vi "XML_AppendSubContent.vi"(10 "string":string, 11 "XML String":string) -> (3 "delimited string":string)   [LabVIEW 2014]
uses:
  <userlib>/_OpenG.lib/string/string.llb/Trim Whitespace (String Array)__ogtk.vi
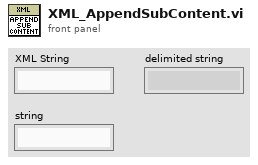
[diagram p1: front panel]
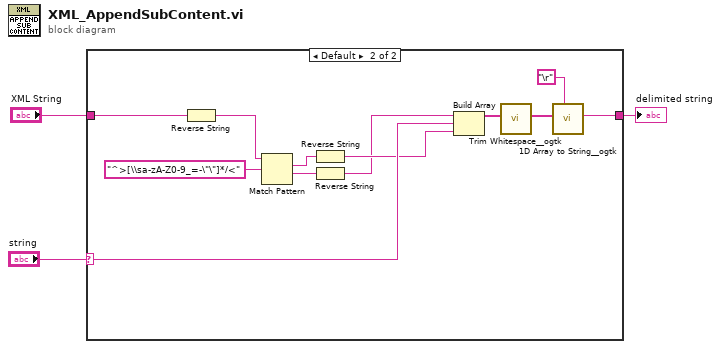
[diagram p0: block diagram]
diagram:
  n1 = case shown="Default" "string" {
    selector: "string" -> [_ w11]
    tunnel: [w4 w14] -> w3
    tunnel: "XML String" -> [w4 w13]
    frame "" {
    }
    frame Default {
      n2 = Reverse String(1:w13) -> (0:w8:string)
      n3 = Match Pattern(string=w8, regular expression="^>[\\sa-zA-Z0-9_=-\"\"]*/<" ("string")) -> (match substring=w5:string, after substring=w12:string)  [unwired: 1 in, 2 out]
      n4 = Reverse String(1:w5) -> (0:w10:string)
      n5 = Reverse String(1:w12) -> (0:w9:string)
      n6 = Build Array(w9, w11, w10) -> (w6:string[])
      n7 = call-poly <userlib>:"Trim Whitespace__ogtk.vi"("String in"=w6) -> ("String out"=w16:string[])  [unwired: 6 in]
      n8 = call <userlib>:"1D Array to String__ogtk.vi"("delimiter (Tab)"="\r", "Array of Strings"=w16) -> ("delimited string"=w14:string)  [unwired: 9 in]
    }
  }
  "delimited string" <- w3
